vi "Periodic Tasks.vi"(8 "error in":errorcluster) -> ()   [LabVIEW 2020]
doc: "This VI runs in parallel to other tasks. It can contain as many user-defined periodic loops as you need. These can carry out PID or other sorts of timed response."
uses:
  <vilib>/Rock Robotics/WPI/Utilities/WPI_GetSetVariantRefNum.vi
  <vilib>/Rock Robotics/Network Tables/NT Read Number.vi
  Robot Global Data.vi
panel:
  # "t"
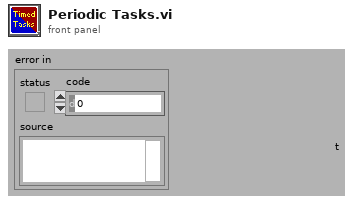
[diagram p1: front panel]
types:
  T1 = typedef "WPI_RobotDriveDevRef.ctl" = cluster{"DevStatus":errorcluster, "Motors[]":T2[], "Square Inputs":bool, "Max Output":dbl}
  T2 = typedef "WPI_MotorControlDeviceRef.ctl" = cluster{"DeviceStatus":errorcluster, "Type":T3, "PWM":cluster{"PWM Channel":T4, "DeadBand":T5}, "CAN":cluster{"Device Number":u8, "SetOutput VI Ref":variant, "GetOutput VI Ref":variant, "Enable VI Ref":variant, "Disable VI Ref":variant, "Data":variant}, "Invert":bool, "DIO PWM":cluster{"PWM \"Enable\" Channel":T4, "DIOChannel":T6, "PWM Rate":dbl}}
  T3 = typedef "WPI_MotorControlType.ctl" = enum16{"PWM", "CAN", "DIO PWM"}
  T4 = typedef "FPGA_DIOPWMChannel.ctl" = enum8{"PWM 0", "PWM 1", "PWM 2", "PWM 3", "PWM 4", "PWM 5", "PWM 6", "PWM 7", "PWM 8", "PWM 9", "PWM MXP 0", "PWM MXP 1", "PWM MXP 2", "PWM MXP 3", "PWM MXP 4", "PWM MXP 5", "PWM MXP 6", "PWM MXP 7", "PWM MXP 8", "PWM MXP 9", "Invalid"}
  T5 = typedef "WPI_PWMDeadband.ctl" = cluster{"Name":string, "maxPositivePwm":i32, "minPositivePwm":i32, "centerPwm":i32, "maxNegativePwm":i32, "minNegativePwm":i32, "angularRange":u16}
  T6 = typedef "FPGA_DIOChannel.ctl" = enum8{"DIO 0", "DIO 1", "DIO 2", "DIO 3", "DIO 4", "DIO 5", "DIO 6", "DIO 7", "DIO 8", "DIO 9", "DIO MXP 0", "DIO MXP 1", "DIO MXP 2", "DIO MXP 3", "DIO MXP 4", "DIO MXP 5", "DIO MXP 6", "DIO MXP 7", "DIO MXP 8", "DIO MXP 9", "DIO MXP 10", "DIO MXP 11", "DIO MXP 12", "DIO MXP 13", "DIO MXP 14", "DIO MXP 15", "SPI Port CS1", "SPI Port CS2", "SPI Port CS3", "SPI Port MISO", "SPI Port MOSI", "Invalid"}
  T7 = typedef "WPI_JoystickDevRef.ctl" = cluster{"Device":T8}
  T8 = typedef "WPI_JoystickDeviceEnum.ctl" = enum16{"USB 0", "USB 1", "USB 2", "USB 3", "USB 4", "USB 5"}
  T9 = cluster{"JoystickDevRef":T7, "RobotDriveDevRef":T1, "Numeric":dbl, "Numeric":dbl}
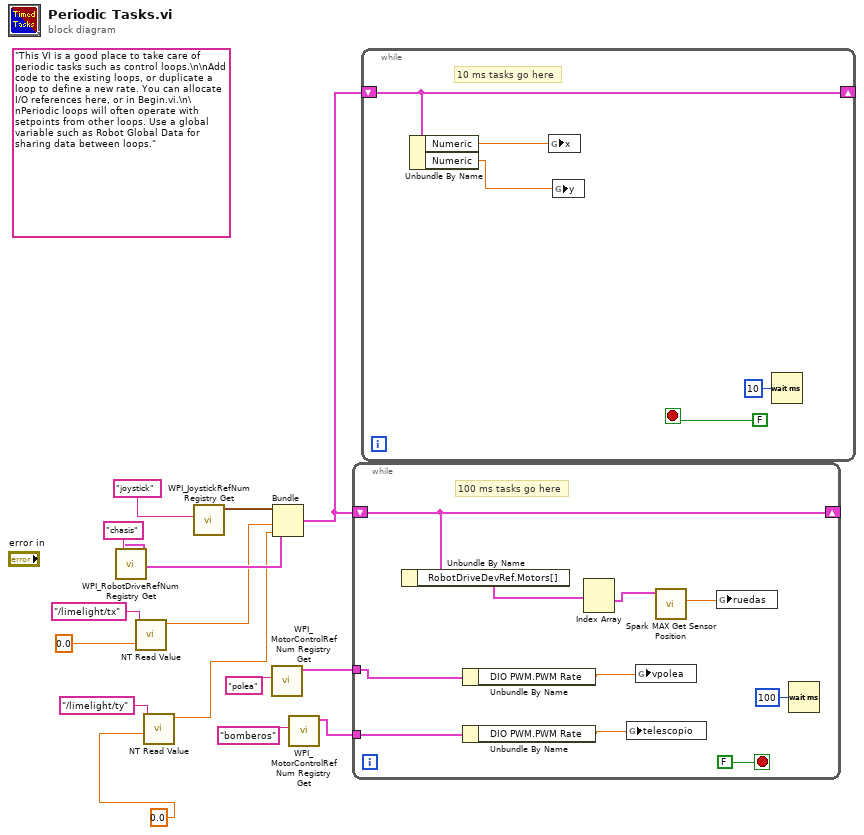
[diagram p0: block diagram]
diagram:
  (unwired) "This VI is a good place to take care of periodic tasks such as control loops.\n\nAdd code to the existing loops, or duplicate a loop to define a new rate. You can allocate I/O references here, or in Begin.vi.\n\nPeriodic loops will often operate with setpoints from other loops. Use a global variable such as Robot Global Data for sharing data between loops."
  n1 = call <vilib>:"WPI_RobotDriveRefNum Registry Get.vi"("refnum name"="chasis") -> ("RobotDriveDevRef"=w12:T1)  [unwired: 1 in, 9 out]
  n2 = call-poly <vilib>:"NT Read Value.vi"("Default Value"=0.0, "Name"="/limelight/tx") -> ("Numeric"=w4:dbl)  [unwired: 8 in, 1 out]
  n3 = call-poly <vilib>:"NT Read Value.vi"("Default Value"=0.0, "Name"="/limelight/ty") -> ("Numeric"=w3:dbl)  [unwired: 8 in, 1 out]
  n4 = call <vilib>:"WPI_JoystickRefNum Registry Get.vi"("refnum name"="joystick") -> ("JoystickDevRef"=w13:T7)  [unwired: 1 in, 9 out]
  n5 = call <vilib>:"WPI_MotorControlRefNum Registry Get.vi"("refnum name"="polea") -> ("MotorControlDevRef"=w9:T2)  [unwired: 9 in, 1 out]
  n6 = Bundle("JoystickDevRef"=w13, "RobotDriveDevRef"=w12, "Numeric"=w4, "Numeric"=w3) -> (w11:T9)  [unwired: 1 out]
  n7 = call <vilib>:"WPI_MotorControlRefNum Registry Get.vi"("refnum name"="bomberos") -> ("MotorControlDevRef"=w1:T2)  [unwired: 9 in, 1 out]
  n8 = while {
    shift-right: [w20] -> _
    shift-left: w11 -> [w20]
    tunnel: w9 -> [w19]
    tunnel: w1 -> [w16]
    stop <- FALSE stop-if-true
    # "100 ms tasks go here"
    n9 = Unbundle By Name(w20) -> ("RobotDriveDevRef.Motors[]"=w23:T2[])
    n10 = Unbundle By Name(w19) -> ("DIO PWM.PWM Rate"=w18:dbl)
    n11 = Unbundle By Name(w16) -> ("DIO PWM.PWM Rate"=w17:dbl)
    n12 = Index Array(array=w23) -> (element #1=w22:T2)  [unwired: 2 in, 1 out]
    n13 = global write "Robot Global Data.vi" "telescopio"(w17) -> ()
    n14 = global write "Robot Global Data.vi" "vpolea"(w18) -> ()
    n15 = call <vilib>:"Spark MAX Get Sensor Position.vi"("MotorControlDevRef in"=w22) -> ("Sensor Position"=w21:dbl)  [unwired: 7 in, 3 out]
    n16 = global write "Robot Global Data.vi" "ruedas"(w21) -> ()
    n17 = Wait (ms)(milliseconds to wait=u32 100) -> ()  [unwired: 1 out]
  }
  n18 = while {
    shift-right: [w28] -> _
    shift-left: w11 -> [w28]
    stop <- FALSE stop-if-true
    # "10 ms tasks go here"
    n19 = Unbundle By Name(w28) -> ("Numeric"=w27:dbl, "Numeric"=w26:dbl)
    n20 = global write "Robot Global Data.vi" "x"(w27) -> ()
    n21 = global write "Robot Global Data.vi" "y"(w26) -> ()
    n22 = Wait (ms)(milliseconds to wait=u32 10) -> ()  [unwired: 1 out]
  }
